vi "Click Peak SPL demo.vi"(0 "Pulse Train Params":T1={"Pulse width (us)"=100.0, "Pulse rate (Hz)"=0.0, "Gap (ms)"=0.0, "Polarity"=enum."POS", "PT State"={"Template"=[], "Nperiod"=0, "Index"=0, "Pulse Rate (Hz)"=0.0, "Phase (cycles)"=0.0, "Noff"=0}, "Asynch"=FALSE}, 12 "Sampling Rate (Hz)":dbl, 13 "Npts":i32) -> (6 "Max Level":dbl)   [LabVIEW 2015]
uses:
  Waveform VIs/Pulse Train VIs/Pulse Train Params.ctl
  Waveform VIs/Pulse Train VIs/Pulse Polarity.ctl
  Waveform VIs/Pulse Train VIs/PT-Continuous State.ctl
  <vilib>/Analysis/2dsp.llb/Inverse Real FFT.vi
  Utility VIs/Math VIs/dB to Linear (scalar).vi
  Utility VIs/Math VIs/Linear to dB (scalar).vi
  <vilib>/Analysis/NI_AALPro.lvlib
panel:
  in  "Cal mic sens":dbl
  in  "Cal mic gain":dbl
  out "Waveform Graph 2":dbl[](graph)
  out "Waveform Graph":dbl[](graph)
  in  "Cal File":path
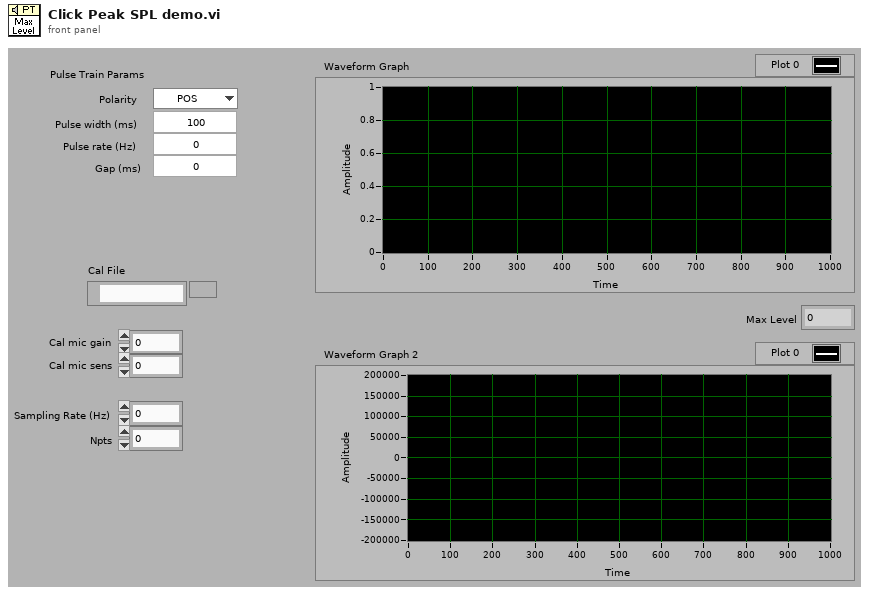
[diagram p1: front panel]
types:
  T1 = typedef "Pulse Train Params.ctl" = cluster{"Pulse width (us)":dbl, "Pulse rate (Hz)":dbl, "Gap (ms)":dbl, "Polarity":T2, "PT State":T3, "Asynch":bool}
  T2 = typedef "Pulse Polarity.ctl" = enum16{"POS", "NEG", "POS-NEG", "NEG-POS"}
  T3 = typedef "PT-Continuous State.ctl" = cluster{"Template":dbl[], "Nperiod":i32, "Index":i32, "Pulse Rate (Hz)":dbl, "Phase (cycles)":dbl, "Noff":i32}
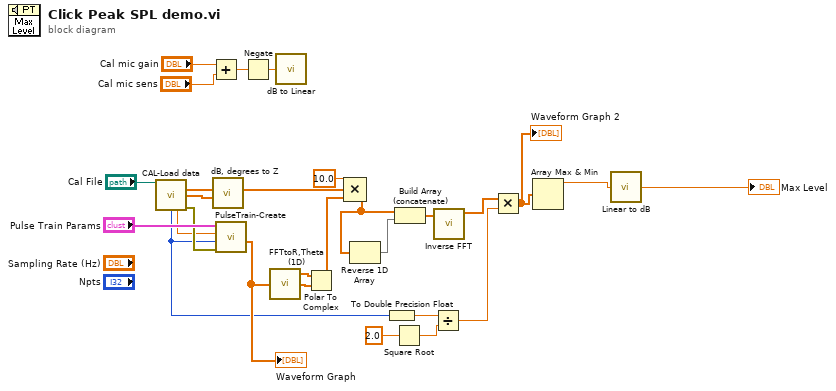
[diagram p0: block diagram]
diagram:
  n1 = call "CAL-Load data.vi"("user path"="Cal File") -> ("Mag"=w26:dbl[], "Phase"=w25:dbl[], "npts"=w10:i32, "Fs (Hz)"=w23:dbl, "error out"=w24:errorcluster)  [unwired: 7 in, 3 out]
  n2 = Add(x="Cal mic gain", y="Cal mic sens") -> (x+y=w16:dbl)
  n3 = call "dB, degrees to Z.vi"("Magnitude (dB)"=w26, "Phase (degrees)"=w25) -> ("Z"=w5:cdb[])  [unwired: 5 in]
  n4 = call "PulseTrain-Create.vi"("error in (no error)"=w24, "Npts"=w10, "Sampling Rate (Hz)"=w23, "Pulse Train Params"="Pulse Train Params") -> ("Waveform"=w19:dbl[])  [unwired: 4 in, 3 out]
  "Waveform Graph" <- w19
  n5 = Negate(x=w16) -> (-x=w15:dbl)
  n6 = call "FFTtoR,Theta (1D).VI"("X"=w19) -> ("+Freq. Mag of FFT"=w21:dbl[], "+Freq Theta of FFT"=w22:dbl[])  [unwired: 1 in]
  n7 = call-poly "dB to Linear.vi"("dB"=w15) -> ()  [unwired: 1 out]
  n8 = Polar To Complex(1:w22, 2:w21) -> (0:w4:cdb[])
  n9 = Compound Arithmetic op=MULTIPLY(10.0, w5, w4) -> (w3:cdb[])
  n10 = Reverse 1D Array(array=w3) -> (reversed array=w14:cdb[])
  n11 = To Double Precision Float(number=w10) -> (double precision float=w9:dbl)
  n12 = Square Root(x=2.0) -> (sqrt(x)=w7:dbl)
  n13 = Build Array (concatenate)(w3, w14) -> (w13:cdb[])
  n14 = Divide(x=w9, y=w7) -> (x/y=w8:dbl)
  n15 = call-poly <vilib>:"Inverse FFT.vi"("FFT {X}"=w13) -> ("X"=w12:dbl[])  [unwired: 9 in, 1 out]
  n16 = Multiply(x=w12, y=w8) -> (x*y=w11:dbl[])
  "Waveform Graph 2" <- w11
  n17 = Array Max & Min(array=w11) -> (max value=w2:dbl)  [unwired: 3 out]
  n18 = call-poly "Linear to dB.vi"("Linear"=w2) -> ("dB"=→"Max Level":dbl)
